vi "GetContainedPathSet.vi"(8 "error in (no error)":errorcluster, 11 "CLabVIEWItem in":refnum<class "CLabVIEWItem.lvclass">) -> (0 "error out":errorcluster, 1 "Contained":set{string}(c389), 3 "CLabVIEWItem out":refnum<class "CLabVIEWItem.lvclass">)   [LabVIEW 2020, in "LabVIEWItem.lvlib" / "CLabVIEWItem.lvclass"]
uses:
  CLabVIEWItem.lvclass
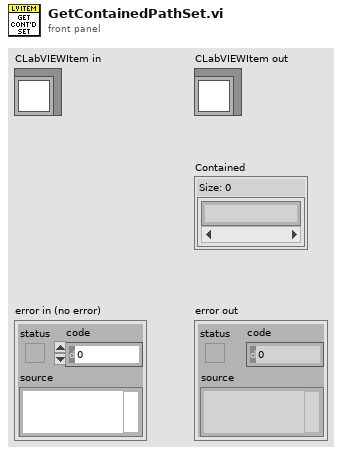
[diagram p1: front panel]
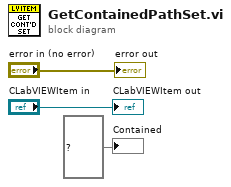
[diagram p0: block diagram]
diagram:
  "error out" <- "error in (no error)"
  "CLabVIEWItem out" <- "CLabVIEWItem in"
  "Contained" <- set{string} {} ("Contained")
